vi "Run Command.vi"(3 "Values":T1(array[cluster]), 4 "Line Index In":i32, 5 "Script":string) -> (0 "Values out":T1(array[cluster]), 1 "Line Index Out":i32, 2 "Done":bool)   [LabVIEW 2017, in "Apple script.lvlib"]
doc: "Looks at a line and runs the appropriate command. Add new commands to this vi."
uses:
  Apple script.lvlib
  Robot Global Data.vi
  Pigeon Gyro.vi
  <vilib>/Rock Robotics/Network Tables/NT Write Value.vi
  <vilib>/Rock Robotics/Network Tables/NT Write Numeric Array.vi
  <vilib>/addons/control/pid/pid.llb/PID.vi
  <vilib>/addons/control/pid/pid.llb/PID (DBL).vi
  Angle Distance.vi
  Parse Number.vi
  Timer.vi
  Parse Subcommand.vi
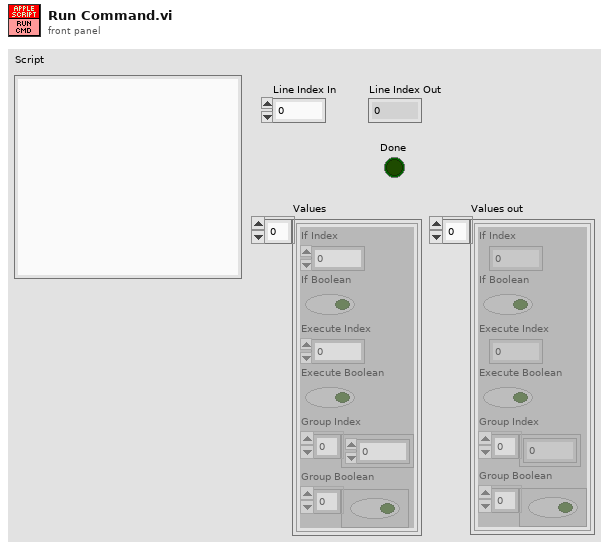
[diagram p1: front panel]
types:
  T1 = cluster{"If Index":i32, "If Boolean":bool, "Execute Index":i32, "Execute Boolean":bool, "Group Index":i32[], "Group Boolean":bool[]}[]
  T2 = cluster{"If Index":i32, "If Boolean":bool, "Execute Index":i32, "Execute Boolean":bool, "Group Index":i32[], "Group Boolean":bool[]}
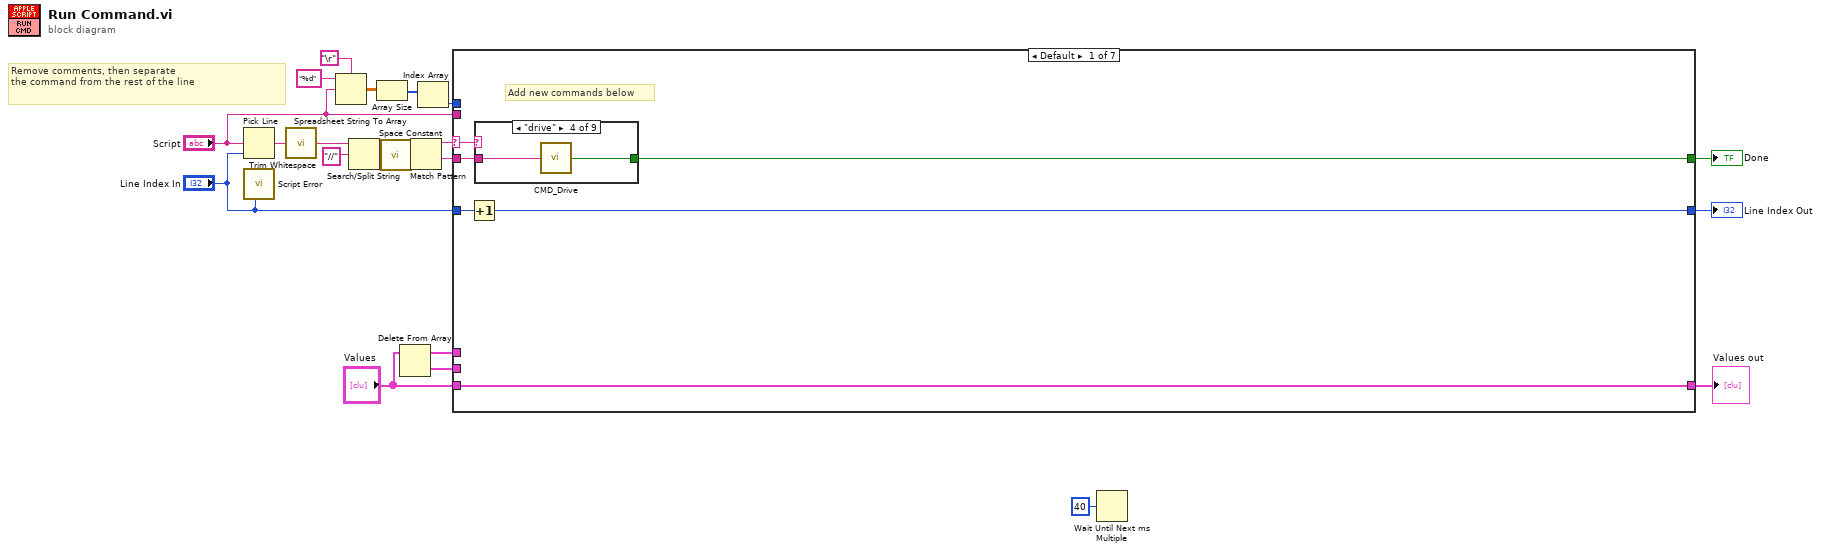
[diagram p0: block diagram]
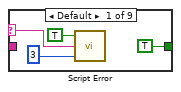
[diagram p2: hidden frame]
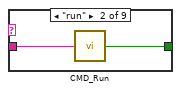
[diagram p3: hidden frame]
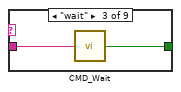
[diagram p4: hidden frame]
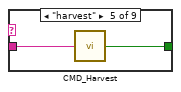
[diagram p5: hidden frame]
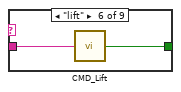
[diagram p6: hidden frame]
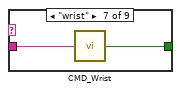
[diagram p7: hidden frame]
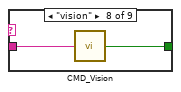
[diagram p8: hidden frame]
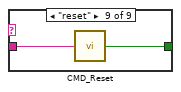
[diagram p9: hidden frame]
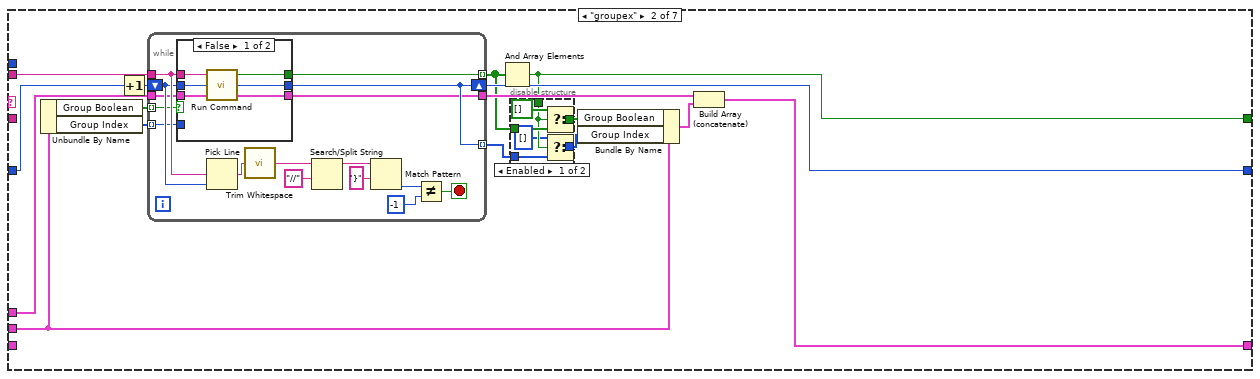
[diagram p10: hidden frame]
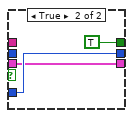
[diagram p12: hidden frame]
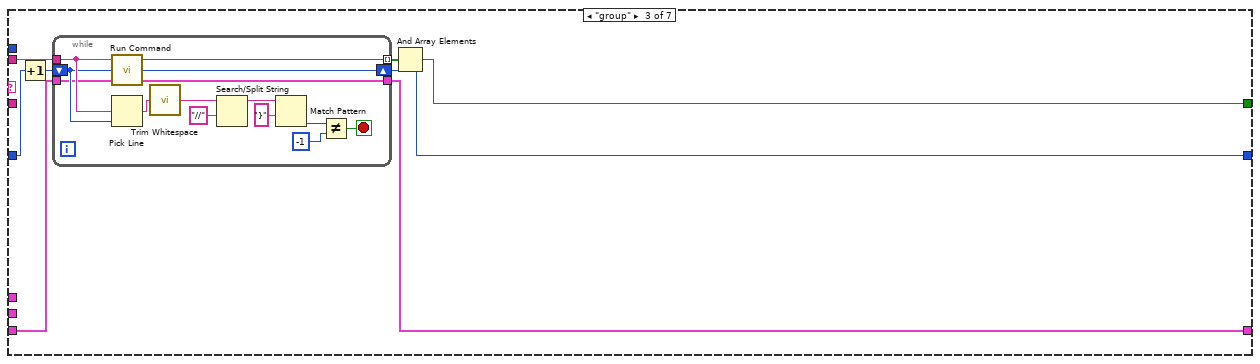
[diagram p13: hidden frame]
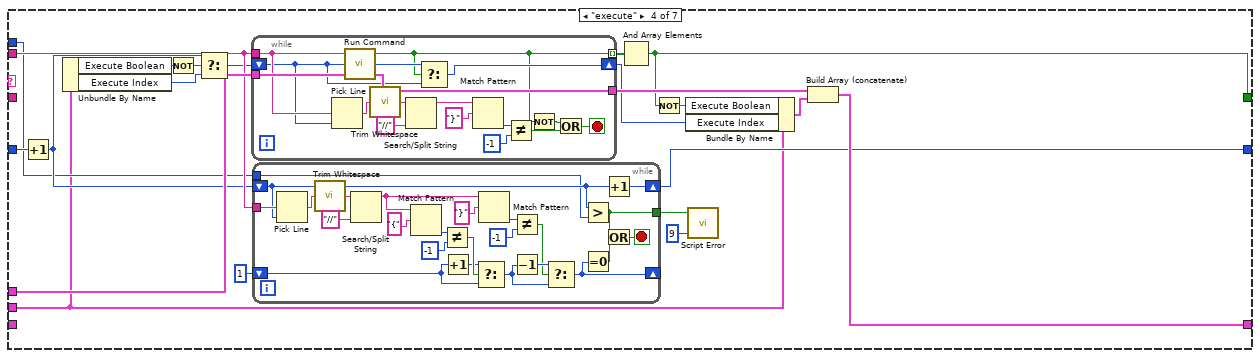
[diagram p14: hidden frame]
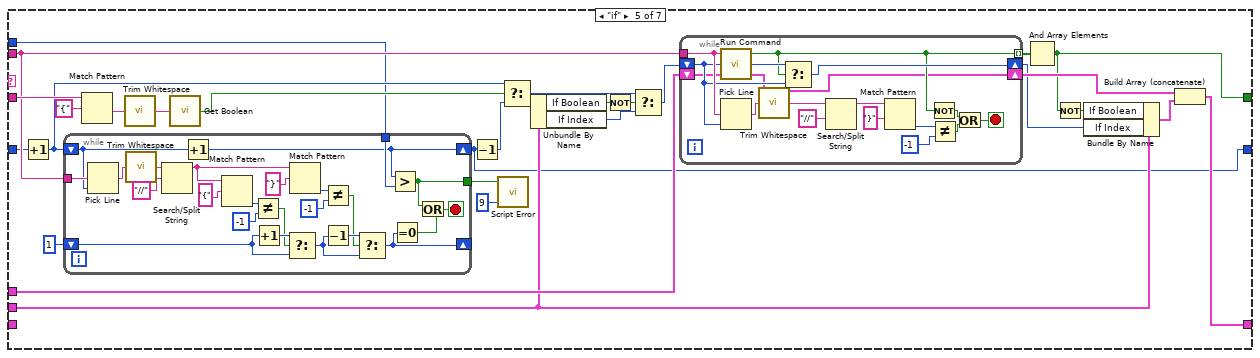
[diagram p15: hidden frame]
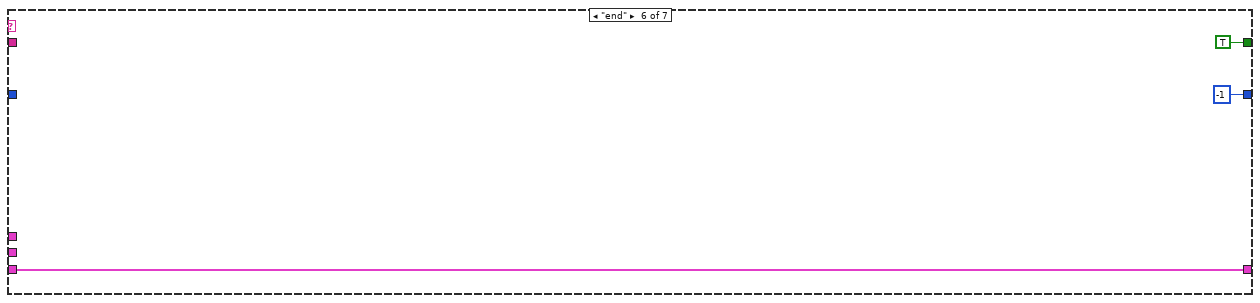
[diagram p16: hidden frame]
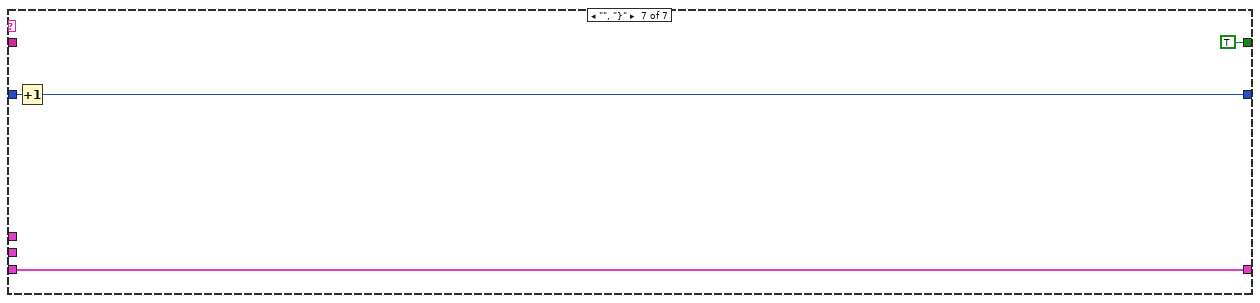
[diagram p17: hidden frame]
diagram:
  # "Remove comments, then separate\nthe command from the rest of the line"
  n1 = Pick Line(multi-line string="Script", line index="Line Index In") -> (output string=w19:string)  [unwired: 1 in]
  n2 = call "Script Error.vi"("Line Number"="Line Index In") -> ()  [unwired: 4 in, 1 out]
  n3 = call <vilib>:"Trim Whitespace.vi"("string"=w19) -> ("trimmed string"=w17:string)  [unwired: 1 in]
  n4 = Spreadsheet String To Array(delimiter (Tab)="\r", format string="%d", spreadsheet string="Script") -> (array=w7:dbl[][])  [unwired: 1 in]
  n5 = Search/Split String(string=w17, search string/char (-)="//") -> (substring before match=w16:string)  [unwired: 1 in, 2 out]
  n6 = Array Size(array=w7) -> (size(s)=w4:i32[])
  n7 = call <vilib>:"Space Constant.vi"() -> ("String"=w21:string)
  n8 = Delete From Array(array="Values") -> (deleted portion=w8:T2, array with subset deleted=w9:T1)  [unwired: 2 in]
  n9 = Match Pattern(string=w16, regular expression=w21) -> (before substring=w15:string, after substring=w14:string)  [unwired: 1 in, 2 out]
  n10 = Index Array(array=w4) -> (element=w2:i32)  [unwired: 1 in]
  n11 = case shown="Default" w15 {
    selector: w15 -> [w25 _ _ _ _ _ _]
    tunnel: "Script" -> [_ w63 w105 w129 w194 _ _]
    tunnel: "Line Index In" -> [w27 w61 w103 w140 w186 _ w255]
    tunnel: [w24 w48 w100 w127 w189 TRUE ("Running") TRUE ("Running")] -> w13
    tunnel: [w26 w62 w104 w126 w182 -1 ("Line Index Out") w254] -> w12
    tunnel: w14 -> [w23 _ _ _ w200 _ _]
    tunnel: "Values" -> [w22 _ w98 _ _ w250 w253]
    tunnel: [w22 w54 w99 w133 w201 w250 w253] -> w11
    tunnel: w9 -> [_ w59 _ w138 w204 _ _]
    tunnel: w8 -> [_ w55 _ w120 w188 _ _]
    tunnel: w2 -> [_ _ _ w122 w185 _ _]
    frame Default {
      # "Add new commands below"
      n12 = Increment(x=w27) -> (x+1=w26:i32)
      n13 = case shown="\"drive\"" w25 {
        selector: w25 -> [w28 _ _ _ _ _ _ _ _]
        tunnel: [TRUE w32 w35 w36 w38 w40 w42 w44 w46] -> w24
        tunnel: w23 -> [_ w33 w34 w37 w39 w41 w43 w45 w47]
        frame Default {
          n14 = call "Script Error.vi"("Error?"=TRUE, "Error Details"=w28, "Error Code"=3) -> ()  [unwired: 2 in, 1 out]
        }
        frame "run" {
          n15 = call "CMD_Run.vi"("Line"=w33) -> ("Done"=w32:bool)
        }
        frame "wait" {
          n16 = call "CMD_Wait.vi"("Line"=w34) -> ("Done"=w35:bool)
        }
        frame "drive" {
          n17 = call "CMD_Drive.vi"("Line"=w37) -> ("Done"=w36:bool)
        }
        frame "harvest" {
          n18 = call "CMD_Harvest.vi"("Line"=w39) -> ("Done"=w38:bool)
        }
        frame "lift" {
          n19 = call "CMD_Lift.vi"("Line"=w41) -> ("Done"=w40:bool)
        }
        frame "wrist" {
          n20 = call "CMD_Wrist.vi"("Line"=w43) -> ("Done"=w42:bool)
        }
        frame "vision" {
          n21 = call "CMD_Vision.vi"("Line"=w45) -> ("Done"=w44:bool)
        }
        frame "reset" {
          n22 = call "CMD_Reset.vi"("Line"=w47) -> ("Done"=w46:bool)
        }
      }
    }
    frame "groupex" {
      n23 = Unbundle By Name(w55) -> ("Group Boolean"=w57:bool[], "Group Index"=w51:i32[])
      n24 = Increment(x=w61) -> (x+1=w60:i32)
      n25 = while {
        tunnel: w63 -> [w88]
        tunnel: [w81] -> w52 mode=indexing
        shift-right: [w76] -> w62
        shift-left: w60 -> [w80]
        tunnel: w57 -> [w77] mode=indexing
        tunnel: [w76] -> w56 mode=indexing
        tunnel: w51 -> [w75] mode=indexing
        tunnel: w59 -> [w74]
        tunnel: [w73] -> w58
        stop <- w78 stop-if-true
        n26 = case shown="False" w77 {
          tunnel: w88 -> [w94 _]
          tunnel: [w93 TRUE ("Done")] -> w81
          tunnel: w80 -> [w92 _]
          tunnel: [w91 w96] -> w76
          tunnel: w75 -> [_ w96]
          tunnel: w74 -> [w90 w95]
          tunnel: [w89 w95] -> w73
          frame False {
            n27 = call "Run Command.vi"("Values"=w90, "Line Index In"=w92, "Script"=w94) -> ("Values out"=w89:T1, "Line Index Out"=w91:i32, "Done"=w93:bool)
          }
          frame True {
          }
        }
        n28 = Pick Line(multi-line string=w88, line index=w80) -> (output string=w83:string)  [unwired: 1 in]
        n29 = call <vilib>:"Trim Whitespace.vi"("string"=w83) -> ("trimmed string"=w84:string)  [unwired: 1 in]
        n30 = Search/Split String(string=w84, search string/char (-)="//") -> (substring before match=w79:string)  [unwired: 1 in, 2 out]
        n31 = Match Pattern(string=w79, regular expression="}" ("search string/char (-)")) -> (offset past match=w86:i32)  [unwired: 1 in, 3 out]
        n32 = Not Equal?(x=w86, y=-1) -> (x != y?=w78:bool)
      }
      n33 = And Array Elements(Boolean array=w52) -> (logical AND=w48:bool)
      n34 = disable-structure shown="Enabled" {
        disable-tunnel: w56 -> [w70 w71]
        disable-tunnel: [w69 w72] -> w53
        disable-tunnel: w52 -> [w68 w72]
        disable-tunnel: [w66 w71] -> w50
        disable-tunnel: w48 -> [w65 _]
        frame Enabled {
          n35 = Select(t=bool[] [], s=w65, f=w68) -> (s? t:f=w69:bool[])
          n36 = Select(t=i32[] [], s=w65, f=w70) -> (s? t:f=w66:i32[])
        }
        frame Disabled {
        }
      }
      n37 = Bundle By Name(cluster=w55, "Group Boolean"=w53, "Group Index"=w50) -> (w49:T2)
      n38 = Build Array (concatenate)(w58, w49) -> (w54:T1)
    }
    frame "group" {
      n39 = Increment(x=w103) -> (x+1=w102:i32)
      n40 = while {
        tunnel: w105 -> [w119]
        tunnel: [w112] -> w101 mode=indexing
        shift-right: [w108] -> w104
        shift-left: w102 -> [w111]
        tunnel: w98 -> [w107]
        tunnel: [w106] -> w99
        stop <- w109 stop-if-true
        n41 = call "Run Command.vi"("Values"=w107, "Line Index In"=w111, "Script"=w119) -> ("Values out"=w106:T1, "Line Index Out"=w108:i32, "Done"=w112:bool)
        n42 = Pick Line(multi-line string=w119, line index=w111) -> (output string=w114:string)  [unwired: 1 in]
        n43 = call <vilib>:"Trim Whitespace.vi"("string"=w114) -> ("trimmed string"=w115:string)  [unwired: 1 in]
        n44 = Search/Split String(string=w115, search string/char (-)="//") -> (substring before match=w110:string)  [unwired: 1 in, 2 out]
        n45 = Match Pattern(string=w110, regular expression="}" ("search string/char (-)")) -> (offset past match=w117:i32)  [unwired: 1 in, 3 out]
        n46 = Not Equal?(x=w117, y=-1) -> (x != y?=w109:bool)
      }
      n47 = And Array Elements(Boolean array=w101) -> (logical AND=w100:bool)
    }
    frame "execute" {
      n48 = Increment(x=w140) -> (x+1=w125:i32)
      n49 = Unbundle By Name(w120) -> ("Execute Boolean"=w136:bool, "Execute Index"=w137:i32)
      n50 = Not(x=w136) -> (.not. x?=w132:bool)
      n51 = Select(t=w125, s=w132, f=w137) -> (s? t:f=w124:i32)
      n52 = while {
        tunnel: w129 -> [w169]
        tunnel: [w168] -> w139 mode=indexing
        shift-right: [w179] -> w128
        shift-left: w124 -> [w165]
        tunnel: w138 -> [w178]
        tunnel: [w177] -> w134
        stop <- w181 stop-if-true
        n53 = Pick Line(multi-line string=w169, line index=w165) -> (output string=w173:string)  [unwired: 1 in]
        n54 = call "Run Command.vi"("Values"=w178, "Line Index In"=w165, "Script"=w169) -> ("Values out"=w177:T1, "Line Index Out"=w180:i32, "Done"=w168:bool)
        n55 = call <vilib>:"Trim Whitespace.vi"("string"=w173) -> ("trimmed string"=w174:string)  [unwired: 1 in]
        n56 = Search/Split String(string=w174, search string/char (-)="//") -> (substring before match=w170:string)  [unwired: 1 in, 2 out]
        n57 = Select(t=w180, s=w168, f=w165) -> (s? t:f=w179:i32)
        n58 = Match Pattern(string=w170, regular expression="}" ("search string/char (-)")) -> (offset past match=w176:i32)  [unwired: 1 in, 3 out]
        n59 = Not Equal?(x=w176, y=-1) -> (x != y?=w166:bool)
        n60 = Not(x=w168) -> (.not. x?=w167:bool)
        n61 = Or(x=w167, y=w166) -> (x .or. y?=w181:bool)
      }
      n62 = while {
        shift-right: [w158] -> w126
        shift-left: w125 -> [w145]
        shift-right: [w147] -> _
        shift-left: i16 1 -> [w151]
        tunnel: w129 -> [w146]
        tunnel: w122 -> [w144]
        tunnel: [w141] -> w121
        stop <- w142 stop-if-true
        n63 = Pick Line(multi-line string=w146, line index=w145) -> (output string=w161:string)  [unwired: 1 in]
        n64 = call <vilib>:"Trim Whitespace.vi"("string"=w161) -> ("trimmed string"=w162:string)  [unwired: 1 in]
        n65 = Search/Split String(string=w162, search string/char (-)="//") -> (substring before match=w154:string)  [unwired: 1 in, 2 out]
        n66 = Match Pattern(string=w154, regular expression="{" ("search string/char (-)")) -> (offset past match=w155:i32)  [unwired: 1 in, 3 out]
        n67 = Not Equal?(x=w155, y=-1) -> (x != y?=w153:bool)
        n68 = Increment(x=w151) -> (x+1=w152:i16)
        n69 = Select(t=w152, s=w153, f=w151) -> (s? t:f=w149:i16)
        n70 = Match Pattern(string=w154, regular expression="}" ("search string/char (-)")) -> (offset past match=w164:i32)  [unwired: 1 in, 3 out]
        n71 = Not Equal?(x=w164, y=-1) -> (x != y?=w148:bool)
        n72 = Decrement(x=w149) -> (x-1=w150:i16)
        n73 = Select(t=w150, s=w148, f=w149) -> (s? t:f=w147:i16)
        n74 = Greater?(x=w145, y=w144) -> (0:w141:bool)
        n75 = Equal To 0?(x=w147) -> (x = 0?=w143:bool)
        n76 = Increment(x=w145) -> (x+1=w158:i32)
        n77 = Or(x=w141, y=w143) -> (x .or. y?=w142:bool)
      }
      n78 = And Array Elements(Boolean array=w139) -> (logical AND=w127:bool)
      n79 = Not(x=w127) -> (.not. x?=w131:bool)
      n80 = Bundle By Name(cluster=w120, "Execute Boolean"=w131, "Execute Index"=w128) -> (w135:T2)
      n81 = call "Script Error.vi"("Error?"=w121, "Error Code"=9) -> ()  [unwired: 3 in, 1 out]
      n82 = Build Array (concatenate)(w134, w135) -> (w133:T1)
    }
    frame "if" {
      n83 = Increment(x=w186) -> (x+1=w193:i32)
      n84 = while {
        shift-right: [w212] -> w182
        shift-left: w193 -> [w215]
        shift-right: [w218] -> _
        shift-left: 1 -> [w222]
        tunnel: w194 -> [w217]
        tunnel: w185 -> [w213]
        tunnel: [w210] -> w184
        stop <- w211 stop-if-true
        n85 = Pick Line(multi-line string=w217, line index=w215) -> (output string=w229:string)  [unwired: 1 in]
        n86 = call <vilib>:"Trim Whitespace.vi"("string"=w229) -> ("trimmed string"=w230:string)  [unwired: 1 in]
        n87 = Search/Split String(string=w230, search string/char (-)="//") -> (substring before match=w224:string)  [unwired: 1 in, 2 out]
        n88 = Increment(x=w215) -> (x+1=w212:i32)
        n89 = Match Pattern(string=w224, regular expression="{" ("search string/char (-)")) -> (offset past match=w225:i32)  [unwired: 1 in, 3 out]
        n90 = Not Equal?(x=w225, y=-1) -> (x != y?=w216:bool)
        n91 = Increment(x=w222) -> (x+1=w223:i32)
        n92 = Select(t=w223, s=w216, f=w222) -> (s? t:f=w220:i32)
        n93 = Match Pattern(string=w224, regular expression="}" ("search string/char (-)")) -> (offset past match=w232:i32)  [unwired: 1 in, 3 out]
        n94 = Not Equal?(x=w232, y=-1) -> (x != y?=w219:bool)
        n95 = Decrement(x=w220) -> (x-1=w221:i32)
        n96 = Select(t=w221, s=w219, f=w220) -> (s? t:f=w218:i32)
        n97 = Greater?(x=w212, y=w213) -> (0:w210:bool)
        n98 = Equal To 0?(x=w218) -> (x = 0?=w211:bool)
        n99 = Or(x=w210, y=w211) -> ()  [unwired: 1 out]
      }
      n100 = Match Pattern(string=w200, regular expression="{") -> (before substring=w198:string)  [unwired: 1 in, 3 out]
      n101 = call <vilib>:"Trim Whitespace.vi"("string"=w198) -> ("trimmed string"=w197:string)  [unwired: 1 in]
      n102 = call "Get Boolean.vi"("Name"=w197) -> ("Value"=w207:bool)
      n103 = Decrement(x=w182) -> (x-1=w187:i32)
      n104 = call "Script Error.vi"("Error?"=w184, "Error Code"=9) -> ()  [unwired: 3 in, 1 out]
      n105 = Select(t=w193, s=w207, f=w187) -> (s? t:f=w208:i32)
      n106 = Unbundle By Name(w188) -> ("If Boolean"=w206:bool, "If Index"=w205:i32)
      n107 = Not(x=w206) -> (.not. x?=w196:bool)
      n108 = Select(t=w208, s=w196, f=w205) -> (s? t:f=w191:i32)
      n109 = while {
        tunnel: w194 -> [w249]
        tunnel: [w235] -> w209 mode=indexing
        shift-right: [w239] -> w190
        shift-left: w191 -> [w236]
        shift-right: [w233] -> w202
        shift-left: w204 -> [w234]
        stop <- w248 stop-if-true
        n110 = call "Run Command.vi"("Values"=w234, "Line Index In"=w236, "Script"=w249) -> ("Values out"=w233:T1, "Line Index Out"=w237:i32, "Done"=w235:bool)
        n111 = Pick Line(multi-line string=w249, line index=w236) -> (output string=w243:string)  [unwired: 1 in]
        n112 = call <vilib>:"Trim Whitespace.vi"("string"=w243) -> ("trimmed string"=w244:string)  [unwired: 1 in]
        n113 = Select(t=w237, s=w235, f=w236) -> (s? t:f=w239:i32)
        n114 = Search/Split String(string=w244, search string/char (-)="//") -> (substring before match=w238:string)  [unwired: 1 in, 2 out]
        n115 = Match Pattern(string=w238, regular expression="}" ("search string/char (-)")) -> (offset past match=w246:i32)  [unwired: 1 in, 3 out]
        n116 = Not(x=w235) -> (.not. x?=w240:bool)
        n117 = Not Equal?(x=w246, y=-1) -> (x != y?=w241:bool)
        n118 = Or(x=w240, y=w241) -> (x .or. y?=w248:bool)
      }
      n119 = And Array Elements(Boolean array=w209) -> (logical AND=w189:bool)
      n120 = Not(x=w189) -> (.not. x?=w195:bool)
      n121 = Bundle By Name(cluster=w188, "If Boolean"=w195, "If Index"=w190) -> (w203:T2)
      n122 = Build Array (concatenate)(w202, w203) -> (w201:T1)
    }
    frame "end" {
    }
    frame "", "}" {
      n123 = Increment(x=w255) -> (x+1=w254:i32)
    }
  }
  "Line Index Out" <- w12
  "Done" <- w13
  "Values out" <- w11
  n124 = Wait Until Next ms Multiple(millisecond multiple=u32 40 ("milliseconds to wait")) -> ()  [unwired: 1 out]
